vi "ESP100_Device.vi"(7 "Device-specific in":variant, 8 "error in (no error)":errorcluster, 10 "Position in":dbl[](array[numeric]), 11 "Operation":T2(ring)) -> (0 "error out":errorcluster, 1 "Device properties":cluster{"Axes":string[], "Tolerance":dbl[][]}, 2 "Position out":dbl[](array[numeric]), 3 "Status":T1, 5 "Device-specific out":variant)   [LabVIEW 2015]
uses:
  <vilib>/Instr/_visa.llb/VISA Open Access Mode.ctl
  <vilib>/Instr/_visa.llb/VISA Configure Serial Port (Instr).vi
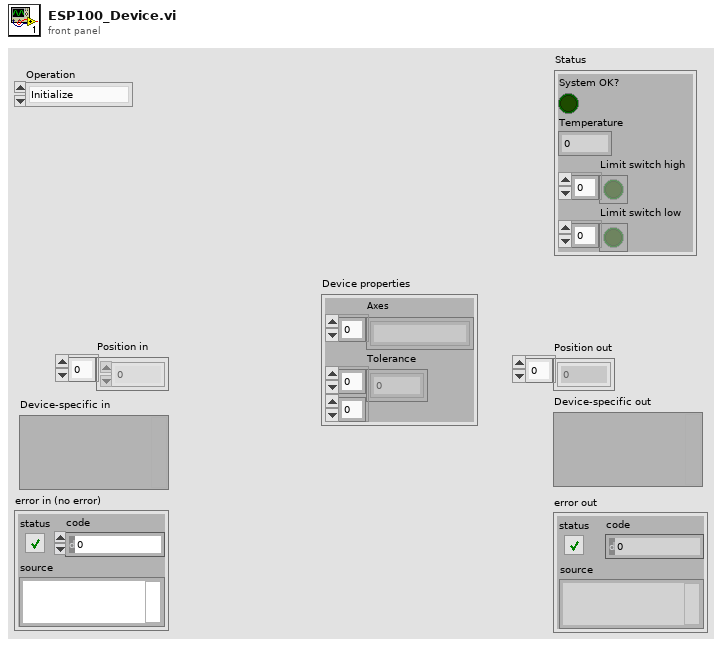
[diagram p1: front panel]
types:
  T1 = cluster{"System OK?":bool, "Temperature":dbl, "Limit switch high":bool[], "Limit switch low":bool[]}
  T2 = enum16{"Initialize", "Shut down", "Set position", "Get position", "Get status", "Other settings"}
  T3 = cluster{"COM port":refnum<visa-resource-name>, "Timeout":u32}
  T4 = typedef "VISA Open Access Mode.ctl" = u32
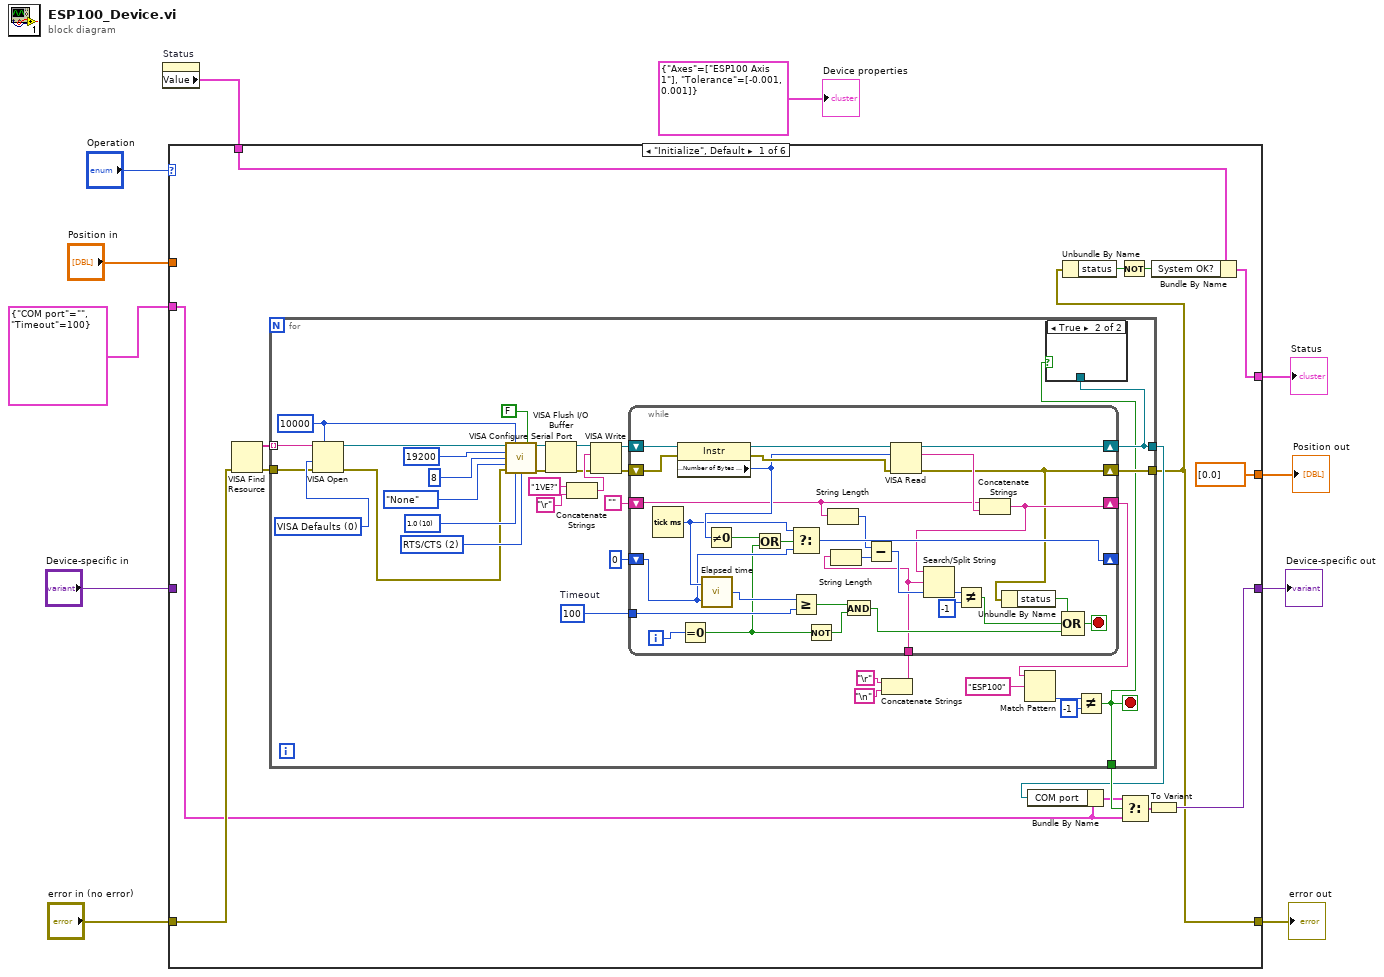
[diagram p0: block diagram]
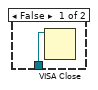
[diagram p2: hidden frame]
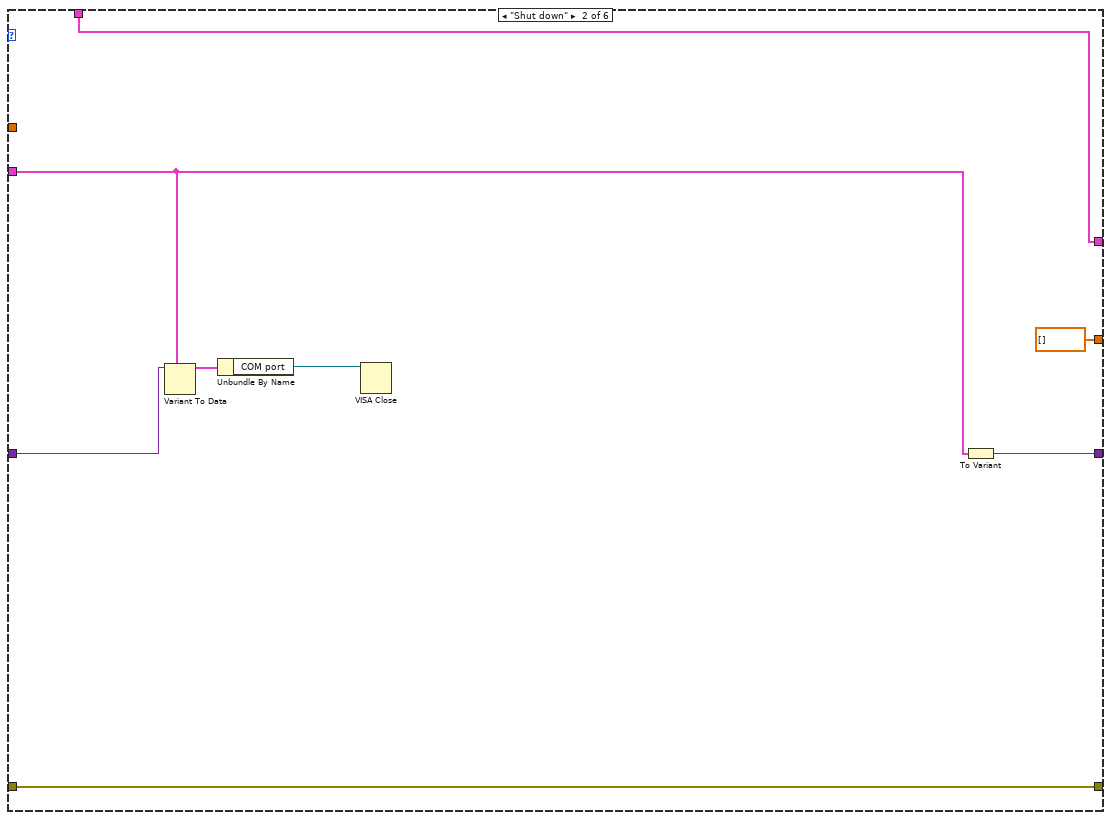
[diagram p3: hidden frame]
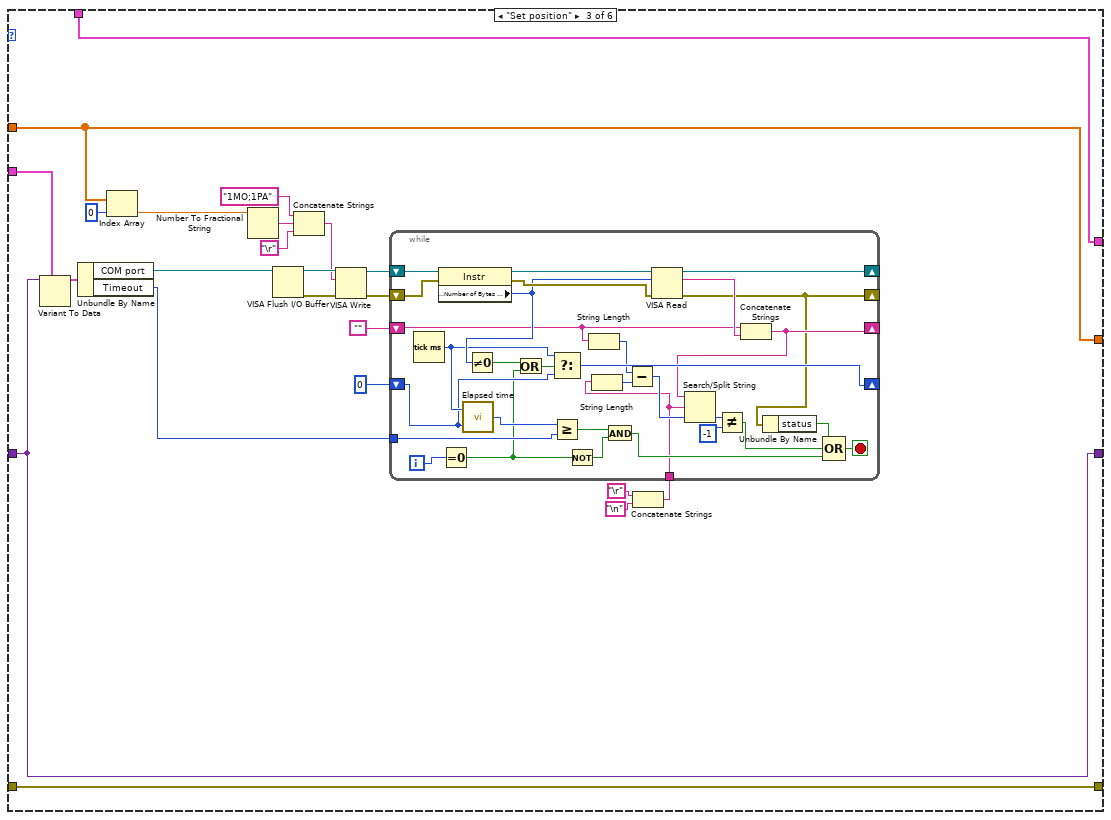
[diagram p4: hidden frame]
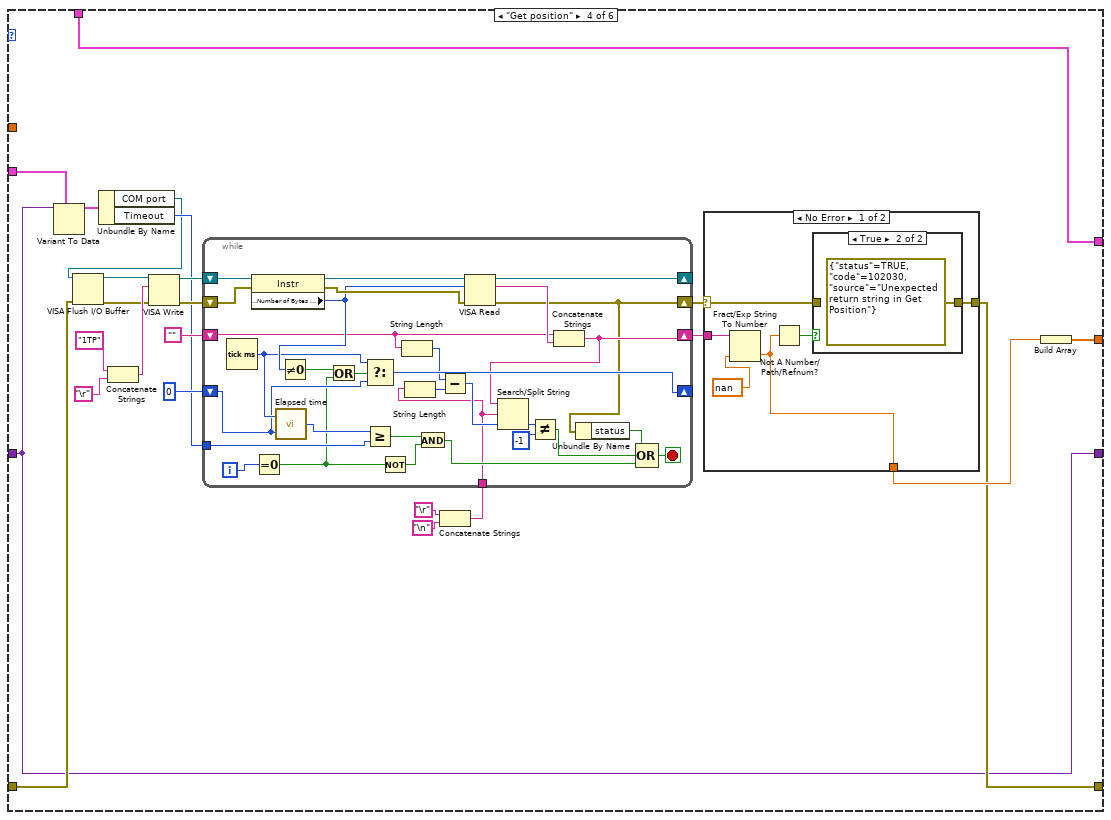
[diagram p5: hidden frame]
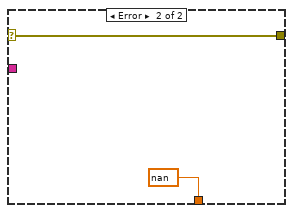
[diagram p7: hidden frame]
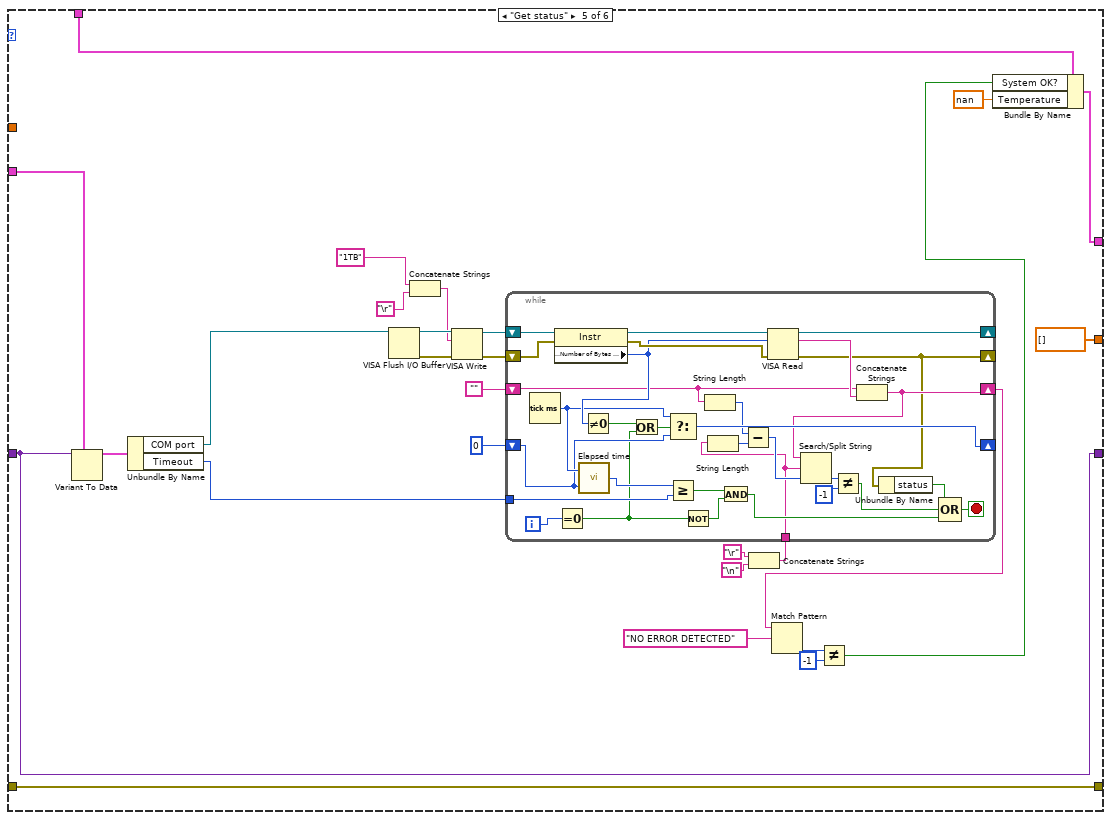
[diagram p8: hidden frame]
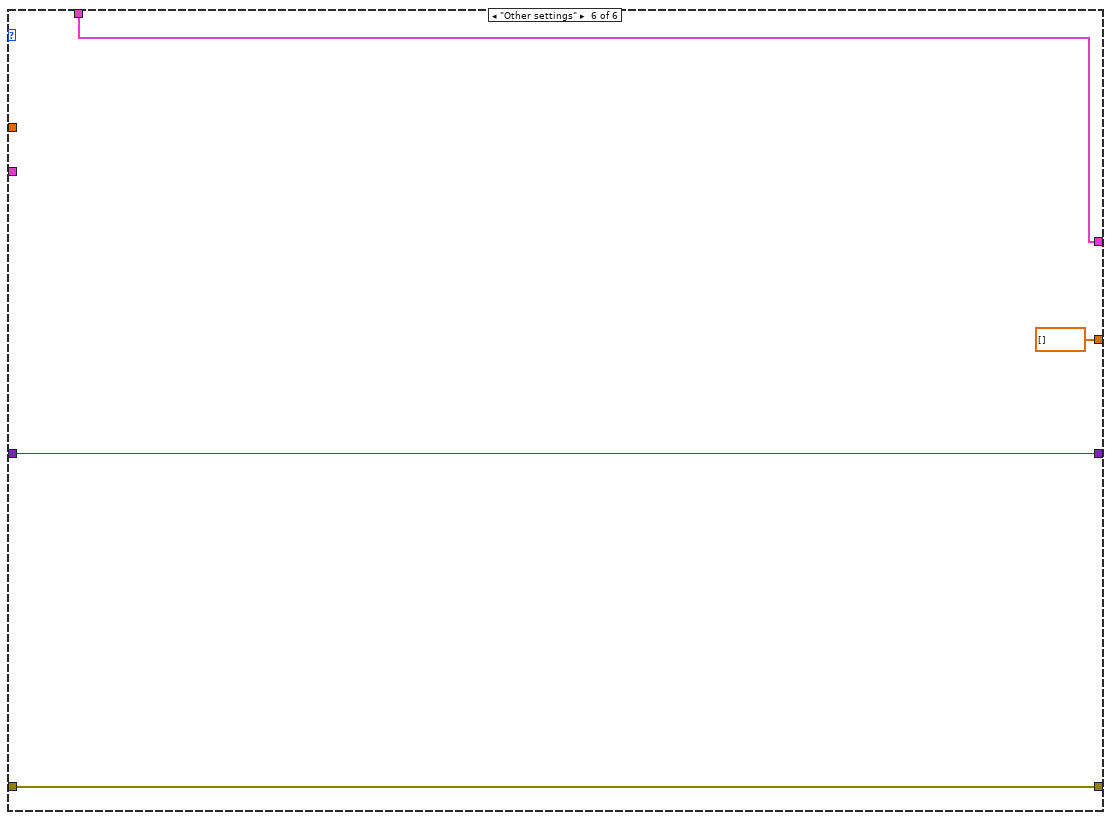
[diagram p9: hidden frame]
diagram:
  n1 = property on="Status" class="Clust (strict)"() -> ("Value"=w10:T1)  [unwired: 2 in, 2 out]
  n2 = case shown="\"Initialize\", Default" "Operation" {
    tunnel: "Position in" -> [_ _ w104 _ _ _]
    tunnel: w10 -> [w26 w100 w123 w178 w246 w281]
    tunnel: [w25 w100 w123 w178 w245 w281] -> w9
    tunnel: "Device-specific in" -> [_ w97 w111 w159 w230 w280]
    tunnel: [dbl[] [0.0] ("Position in") dbl[] [] ("Position in") w104 w162 dbl[] [] ("Position in") dbl[] [] ("Position in")] -> w6
    tunnel: [w18 w94 w111 w159 w230 w280] -> w5
    tunnel: [w15 w99 w122 w161 w243 w279] -> w4
    tunnel: "error in (no error)" -> [w16 w99 w122 w160 w243 w279]
    tunnel: T3 {"COM port"="", "Timeout"=100} -> [w13 w95 w110 w158 w229 _]
    frame "Initialize", Default {
      n3 = VISA Find Resource(8:w16) -> (0:w17:errorcluster, 3:w23:string[])  [unwired: 2 in, 1 out]
      n4 = for {
        tunnel: w23 -> [w50] mode=indexing
        tunnel: [w28] -> w21
        tunnel: [w27] -> w22
        tunnel: w17 -> [w30]
        tunnel: [w29] -> w15
        stop <- w27 stop-if-true
        w40 = u32 100  # Timeout
        w51 = u32 10000 ("timeout (10sec)")
        w53 = T4 0 items=["VISA Defaults"=0, "Exclusive Lock"=1, "Load Configured Settings"=4] ("Access Mode")
        w55 = u16 2 items=["None", "XON/XOFF", "RTS/CTS", "XON/XOFF & RTS/CTS", "DTR/DSR", "XON/XOFF & DTR/DSR"] ("flow control (0:none)")
        w56 = u16 10 items=["1.0"=10, "1.5"=15, "2.0"=20] ("stop bits (10: 1 bit)")
        n5 = VISA Open(timeout (0)=w51, access mode=w53, error in (no error)=w30, VISA resource name=w50) -> (VISA resource name=w54:refnum<visa-resource-name>, error out=w52:errorcluster)  [unwired: 1 in]
        n6 = call-poly "VISA Configure Serial Port"("VISA resource name"=w54, "timeout (10sec)"=w51, "Enable Termination\nChar (T)"=FALSE ("Enable Termination\nChar (T)"), "baud rate (9600)"=u32 19200, "data bits (8)"=u16 8, "parity (0:none)"=enum16{"None", "Odd", "Even", "Mark", "Space"}."None", "error in (no error)"=w52, "stop bits (10: 1 bit)"=w56, "flow control (0:none)"=w55) -> ("VISA resource name out"=w35:refnum<visa-resource-name>, "error out"=w36:errorcluster)  [unwired: 5 in]
        n7 = VISA Flush I/O Buffer(VISA resource name=w35, error in (no error)=w36) -> (VISA resource name out=w48:refnum<visa-resource-name>, error out=w46:errorcluster)  [unwired: 1 in]
        n8 = Concatenate Strings("1VE?", "\r") -> (w47:string)
        n9 = VISA Write(VISA resource name=w48, write buffer=w47, error in (no error)=w46) -> (VISA resource name out=w45:refnum<visa-resource-name>, error out=w44:errorcluster)  [unwired: 1 out]
        n10 = Concatenate Strings("\r", "\n") -> (w37:string)
        n11 = while {
          shift-right: [w88] -> w28
          shift-left: w45 -> [w92]
          shift-right: [w62] -> w29
          shift-left: w44 -> [w91]
          shift-right: [w69] -> w34
          shift-left: "" -> [w68]
          shift-right: [w77] -> _
          shift-left: u32 0 -> [w74]
          tunnel: w40 -> [w75]
          tunnel: w37 -> [w63]
          i -> [w80]
          stop <- w87 stop-if-true
          n12 = Tick Count (ms)() -> (millisecond timer value=w78:u32)
          n13 = property class="Instr"(reference=w92, error in=w91) -> (reference out=w90:refnum<visa-resource-name>, error out=w89:errorcluster, "Serial Settings:Number of Bytes at Serial Port"=w82:u32)
          n14 = Equal To 0?(x=w80) -> (x = 0?=w70:bool)
          n15 = call "Elapsed time.vi"("Start time (ms)"=w74, "Current time (ms)"=w78) -> ("Elapsed time"=w76:u32)
          n16 = Not Equal To 0?(x=w82) -> (x != 0?=w81:bool)
          n17 = Or(x=w81, y=w70) -> (x .or. y?=w79:bool)
          n18 = Select(t=w78, s=w79, f=w74) -> (s? t:f=w77:u32)
          n19 = Greater Or Equal?(x=w76, y=w75) -> (x >= y?=w72:bool)
          n20 = Not(x=w70) -> (.not. x?=w71:bool)
          n21 = String Length(string=w68) -> (length=w66:i32)
          n22 = String Length(string=w63) -> (length=w67:i32)
          n23 = And(x=w72, y=w71) -> (x .and. y?=w73:bool)
          n24 = Subtract(x=w66, y=w67) -> (x-y=w65:i32)
          n25 = VISA Read(VISA resource name=w90, byte count=w82, error in (no error)=w89) -> (VISA resource name out=w88:refnum<visa-resource-name>, read buffer=w86:string, error out=w62:errorcluster)  [unwired: 1 out]
          n26 = Concatenate Strings(w68, w86) -> (w69:string)
          n27 = Search/Split String(string=w69, search string/char (-)=w63, offset (0)=w65) -> (offset of match=w85:i32)  [unwired: 2 out]
          n28 = Not Equal?(x=w85, y=-1) -> (x != y?=w83:bool)
          n29 = Unbundle By Name(w62) -> ("status"=w64:bool)
          n30 = Compound Arithmetic op=OR(w64, w83, w73) -> (w87:bool)
        }
        n31 = Match Pattern(string=w34, regular expression="ESP100" ("y")) -> (offset past match=w32:i32)  [unwired: 1 in, 3 out]
        n32 = Not Equal?(x=w32, y=-1) -> (x != y?=w27:bool)
        n33 = case shown="True" w27 {
          tunnel: w28 -> [w61 _]
          frame False {
            n34 = VISA Close(VISA resource name=w61) -> ()  [unwired: 1 in, 1 out]
          }
          frame True {
          }
        }
      }
      n35 = Bundle By Name(cluster=w13, "COM port"=w21) -> (w20:T3)
      n36 = Unbundle By Name(w15) -> ("status"=w14:bool)
      n37 = Not(x=w14) -> (.not. x?=w12:bool)
      n38 = Select(t=w20, s=w22, f=w13) -> (s? t:f=w19:T3)
      n39 = To Variant(anything=w19) -> (Variant=w18:variant)
      n40 = Bundle By Name(cluster=w26, "System OK?"=w12) -> (w25:T1)
    }
    frame "Shut down" {
      n41 = Variant To Data(type=w95, Variant=w97) -> (data=w96:T3)  [unwired: 1 in, 1 out]
      n42 = Unbundle By Name(w96) -> ("COM port"=w93:refnum<visa-resource-name>)
      n43 = VISA Close(VISA resource name=w93) -> ()  [unwired: 1 in, 1 out]
      n44 = To Variant(anything=w95) -> (Variant=w94:variant)
    }
    frame "Set position" {
      n45 = Variant To Data(type=w110, Variant=w111) -> (data=w109:T3)  [unwired: 1 in, 1 out]
      n46 = Unbundle By Name(w109) -> ("COM port"=w107:refnum<visa-resource-name>, "Timeout"=w108:u32)
      n47 = Index Array(array=w104, index=0) -> (element=w103:dbl)
      n48 = Number To Fractional String(number=w103) -> (F-format string=w105:string)  [unwired: 3 in]
      n49 = VISA Flush I/O Buffer(VISA resource name=w107) -> (VISA resource name out=w121:refnum<visa-resource-name>, error out=w120:errorcluster)  [unwired: 2 in]
      n50 = Concatenate Strings("1MO;1PA", w105, "\r") -> (w101:string)
      n51 = VISA Write(VISA resource name=w121, write buffer=w101, error in (no error)=w120) -> (VISA resource name out=w119:refnum<visa-resource-name>, error out=w118:errorcluster)  [unwired: 1 out]
      n52 = Concatenate Strings("\r", "\n") -> (w112:string)
      n53 = while {
        shift-right: [w150] -> _
        shift-left: w119 -> [w154]
        shift-right: [w124] -> _
        shift-left: w118 -> [w153]
        shift-right: [w131] -> _
        shift-left: "" -> [w130]
        shift-right: [w139] -> _
        shift-left: u32 0 -> [w136]
        tunnel: w108 -> [w137]
        tunnel: w112 -> [w125]
        i -> [w142]
        stop <- w149 stop-if-true
        n54 = Tick Count (ms)() -> (millisecond timer value=w140:u32)
        n55 = property class="Instr"(reference=w154, error in=w153) -> (reference out=w152:refnum<visa-resource-name>, error out=w151:errorcluster, "Serial Settings:Number of Bytes at Serial Port"=w144:u32)
        n56 = Equal To 0?(x=w142) -> (x = 0?=w132:bool)
        n57 = call "Elapsed time.vi"("Start time (ms)"=w136, "Current time (ms)"=w140) -> ("Elapsed time"=w138:u32)
        n58 = Not Equal To 0?(x=w144) -> (x != 0?=w143:bool)
        n59 = Or(x=w143, y=w132) -> (x .or. y?=w141:bool)
        n60 = Select(t=w140, s=w141, f=w136) -> (s? t:f=w139:u32)
        n61 = Greater Or Equal?(x=w138, y=w137) -> (x >= y?=w134:bool)
        n62 = Not(x=w132) -> (.not. x?=w133:bool)
        n63 = String Length(string=w130) -> (length=w128:i32)
        n64 = String Length(string=w125) -> (length=w129:i32)
        n65 = And(x=w134, y=w133) -> (x .and. y?=w135:bool)
        n66 = Subtract(x=w128, y=w129) -> (x-y=w127:i32)
        n67 = VISA Read(VISA resource name=w152, byte count=w144, error in (no error)=w151) -> (VISA resource name out=w150:refnum<visa-resource-name>, read buffer=w148:string, error out=w124:errorcluster)  [unwired: 1 out]
        n68 = Concatenate Strings(w130, w148) -> (w131:string)
        n69 = Search/Split String(string=w131, search string/char (-)=w125, offset (0)=w127) -> (offset of match=w147:i32)  [unwired: 2 out]
        n70 = Not Equal?(x=w147, y=-1) -> (x != y?=w145:bool)
        n71 = Unbundle By Name(w124) -> ("status"=w126:bool)
        n72 = Compound Arithmetic op=OR(w126, w145, w135) -> (w149:bool)
      }
    }
    frame "Get position" {
      n73 = Variant To Data(type=w158, Variant=w159) -> (data=w157:T3)  [unwired: 1 in, 1 out]
      n74 = Unbundle By Name(w157) -> ("COM port"=w155:refnum<visa-resource-name>, "Timeout"=w156:u32)
      n75 = VISA Flush I/O Buffer(VISA resource name=w155, error in (no error)=w160) -> (VISA resource name out=w176:refnum<visa-resource-name>, error out=w174:errorcluster)  [unwired: 1 in]
      n76 = Concatenate Strings("1TP", "\r") -> (w175:string)
      n77 = VISA Write(VISA resource name=w176, write buffer=w175, error in (no error)=w174) -> (VISA resource name out=w173:refnum<visa-resource-name>, error out=w172:errorcluster)  [unwired: 1 out]
      n78 = Concatenate Strings("\r", "\n") -> (w164:string)
      n79 = while {
        shift-right: [w215] -> _
        shift-left: w173 -> [w219]
        shift-right: [w189] -> w167
        shift-left: w172 -> [w218]
        shift-right: [w196] -> w168
        shift-left: "" -> [w195]
        shift-right: [w204] -> _
        shift-left: u32 0 -> [w201]
        tunnel: w156 -> [w202]
        tunnel: w164 -> [w190]
        i -> [w207]
        stop <- w214 stop-if-true
        n80 = Tick Count (ms)() -> (millisecond timer value=w205:u32)
        n81 = property class="Instr"(reference=w219, error in=w218) -> (reference out=w217:refnum<visa-resource-name>, error out=w216:errorcluster, "Serial Settings:Number of Bytes at Serial Port"=w209:u32)
        n82 = Equal To 0?(x=w207) -> (x = 0?=w197:bool)
        n83 = call "Elapsed time.vi"("Start time (ms)"=w201, "Current time (ms)"=w205) -> ("Elapsed time"=w203:u32)
        n84 = Not Equal To 0?(x=w209) -> (x != 0?=w208:bool)
        n85 = Or(x=w208, y=w197) -> (x .or. y?=w206:bool)
        n86 = Select(t=w205, s=w206, f=w201) -> (s? t:f=w204:u32)
        n87 = Greater Or Equal?(x=w203, y=w202) -> (x >= y?=w199:bool)
        n88 = Not(x=w197) -> (.not. x?=w198:bool)
        n89 = String Length(string=w195) -> (length=w193:i32)
        n90 = String Length(string=w190) -> (length=w194:i32)
        n91 = And(x=w199, y=w198) -> (x .and. y?=w200:bool)
        n92 = Subtract(x=w193, y=w194) -> (x-y=w192:i32)
        n93 = VISA Read(VISA resource name=w217, byte count=w209, error in (no error)=w216) -> (VISA resource name out=w215:refnum<visa-resource-name>, read buffer=w213:string, error out=w189:errorcluster)  [unwired: 1 out]
        n94 = Concatenate Strings(w195, w213) -> (w196:string)
        n95 = Search/Split String(string=w196, search string/char (-)=w190, offset (0)=w192) -> (offset of match=w212:i32)  [unwired: 2 out]
        n96 = Not Equal?(x=w212, y=-1) -> (x != y?=w210:bool)
        n97 = Unbundle By Name(w189) -> ("status"=w191:bool)
        n98 = Compound Arithmetic op=OR(w191, w210, w200) -> (w214:bool)
      }
      n99 = case shown="No Error" w167 {
        selector: w167 -> [w183 w188]
        tunnel: w168 -> [w182 _]
        tunnel: [w184 w188] -> w161
        tunnel: [w179 nan] -> w163
        frame No Error {
          n100 = Fract/Exp String To Number(string=w182, default (0 dbl)=nan ("t")) -> (number=w179:dbl)  [unwired: 2 in, 1 out]
          n101 = Not A Number/Path/Refnum?(number/path/refnum=w179) -> (NaN/Path/Refnum?=w180:bool)
          n102 = case shown="True" w180 {
            tunnel: [w185 errorcluster {"status"=TRUE, "code"=102030, "source"="Unexpected return string in Get Position"} ("error IO")] -> w184
            tunnel: w183 -> [w185 _]
            frame False {
            }
            frame True {
            }
          }
        }
        frame Error {
        }
      }
      n103 = Build Array(w163) -> (w162:dbl[])
    }
    frame "Get status" {
      n104 = Variant To Data(type=w229, Variant=w230) -> (data=w228:T3)  [unwired: 1 in, 1 out]
      n105 = Unbundle By Name(w228) -> ("COM port"=w226:refnum<visa-resource-name>, "Timeout"=w227:u32)
      n106 = VISA Flush I/O Buffer(VISA resource name=w226) -> (VISA resource name out=w241:refnum<visa-resource-name>, error out=w240:errorcluster)  [unwired: 2 in]
      n107 = Concatenate Strings("1TB", "\r") -> (w231:string)
      n108 = VISA Write(VISA resource name=w241, write buffer=w231, error in (no error)=w240) -> (VISA resource name out=w239:refnum<visa-resource-name>, error out=w238:errorcluster)  [unwired: 1 out]
      n109 = Concatenate Strings("\r", "\n") -> (w233:string)
      n110 = while {
        shift-right: [w273] -> _
        shift-left: w239 -> [w277]
        shift-right: [w247] -> _
        shift-left: w238 -> [w276]
        shift-right: [w254] -> w225
        shift-left: "" -> [w253]
        shift-right: [w262] -> _
        shift-left: u32 0 -> [w259]
        tunnel: w227 -> [w260]
        tunnel: w233 -> [w248]
        i -> [w265]
        stop <- w272 stop-if-true
        n111 = Tick Count (ms)() -> (millisecond timer value=w263:u32)
        n112 = property class="Instr"(reference=w277, error in=w276) -> (reference out=w275:refnum<visa-resource-name>, error out=w274:errorcluster, "Serial Settings:Number of Bytes at Serial Port"=w267:u32)
        n113 = Equal To 0?(x=w265) -> (x = 0?=w255:bool)
        n114 = call "Elapsed time.vi"("Start time (ms)"=w259, "Current time (ms)"=w263) -> ("Elapsed time"=w261:u32)
        n115 = Not Equal To 0?(x=w267) -> (x != 0?=w266:bool)
        n116 = Or(x=w266, y=w255) -> (x .or. y?=w264:bool)
        n117 = Select(t=w263, s=w264, f=w259) -> (s? t:f=w262:u32)
        n118 = Greater Or Equal?(x=w261, y=w260) -> (x >= y?=w257:bool)
        n119 = Not(x=w255) -> (.not. x?=w256:bool)
        n120 = String Length(string=w253) -> (length=w251:i32)
        n121 = String Length(string=w248) -> (length=w252:i32)
        n122 = And(x=w257, y=w256) -> (x .and. y?=w258:bool)
        n123 = Subtract(x=w251, y=w252) -> (x-y=w250:i32)
        n124 = VISA Read(VISA resource name=w275, byte count=w267, error in (no error)=w274) -> (VISA resource name out=w273:refnum<visa-resource-name>, read buffer=w271:string, error out=w247:errorcluster)  [unwired: 1 out]
        n125 = Concatenate Strings(w253, w271) -> (w254:string)
        n126 = Search/Split String(string=w254, search string/char (-)=w248, offset (0)=w250) -> (offset of match=w270:i32)  [unwired: 2 out]
        n127 = Not Equal?(x=w270, y=-1) -> (x != y?=w268:bool)
        n128 = Unbundle By Name(w247) -> ("status"=w249:bool)
        n129 = Compound Arithmetic op=OR(w249, w268, w258) -> (w272:bool)
      }
      n130 = Match Pattern(string=w225, regular expression="NO ERROR DETECTED" ("Display")) -> (offset past match=w222:i32)  [unwired: 1 in, 3 out]
      n131 = Not Equal?(x=w222, y=-1) -> (x != y?=w220:bool)
      n132 = Bundle By Name(cluster=w246, "System OK?"=w220, "Temperature"=nan) -> (w245:T1)
    }
    frame "Other settings" {
    }
  }
  "Status" <- w9
  "Device-specific out" <- w5
  "error out" <- w4
  "Position out" <- w6
  "Device properties" <- cluster{"Axes":string[], "Tolerance":dbl[][]} {"Axes"=["ESP100 Axis 1"], "Tolerance"=[[-0.001, 0.001]]} ("Device properties")
